vi "Get_Error_Data.vi"(0 "Error_Percentage_F_P":path, 2 "Section_E_P":string, 5 "Key_Max_Error":string, 7 "Key_Min_Error":string, 9 "Create?":bool, 11 "Error_In":errorcluster) -> (4 "Error_Data":dbl, 15 "Error_Out":errorcluster)   [LabVIEW 2021]
uses:
  <vilib>/Utility/config.llb/NI_LVConfig.lvlib
  <vilib>/Utility/config.llb/Read Key (Double).vi
  <vilib>/numeric/Random Number (Range) DBL.vi
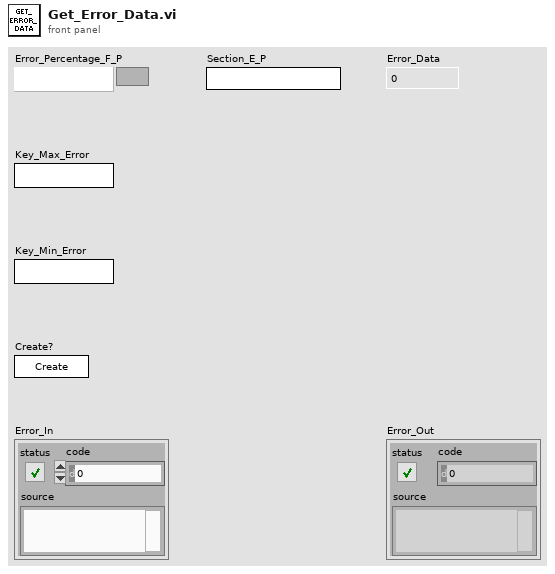
[diagram p1: front panel]
types:
  T1 = typedef "NI_LVConfig.lvlib/Config Data RefNum.ctl" = refnum<k1>
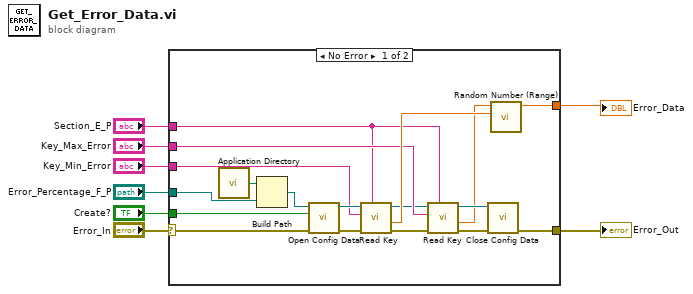
[diagram p0: block diagram]
diagram:
  n1 = case shown="No Error" "Error_In" {
    selector: "Error_In" -> [w9 w27]
    tunnel: "Error_Percentage_F_P" -> [w24 _]
    tunnel: "Create?" -> [w21 _]
    tunnel: [w20 w27] -> w6
    tunnel: [w17 _] -> w5
    tunnel: "Key_Max_Error" -> [w14 _]
    tunnel: "Key_Min_Error" -> [w13 _]
    tunnel: "Section_E_P" -> [w12 _]
    frame No Error {
      n2 = call <vilib>:"Application Directory.vi"() -> ("Application Directory"=w25:path)
      n3 = Build Path(base path=w25, name or relative path=w24) -> (appended path=w26:path)
      n4 = call <vilib>:"Open Config Data.vi"("error in (no error)"=w9, "create file if necessary (T)"=w21, "configuration file path"=w26) -> ("error out"=w22:errorcluster, "refnum"=w23:T1)  [unwired: 6 in, 1 out]
      n5 = call-poly <vilib>:"Read Key.vi"("section"=w12, "error in (no error)"=w22, "key"=w13, "refnum"=w23) -> ("error out"=w11:errorcluster, "value"=w16:dbl, "refnum out"=w10:T1)  [unwired: 4 in, 1 out]
      n6 = call-poly <vilib>:"Read Key.vi"("section"=w12, "error in (no error)"=w11, "key"=w14, "refnum"=w10) -> ("error out"=w19:errorcluster, "value"=w15:dbl, "refnum out"=w18:T1)  [unwired: 4 in, 1 out]
      n7 = call <vilib>:"Close Config Data.vi"("error in (no error)"=w19, "refnum"=w18) -> ("error out"=w20:errorcluster)  [unwired: 8 in, 1 out]
      n8 = call-poly <vilib>:"Random Number (Range).vi"("lower bound (0)"=w16, "upper bound (100)"=w15) -> ("number"=w17:dbl)  [unwired: 9 in]
    }
    frame Error {
    }
  }
  "Error_Out" <- w6
  "Error_Data" <- w5
